vi "EventHandler-String Input with Prompt.vi"(6 "Font":T2={"Normal-Font"={"Name"="Application Font", "Italic"=FALSE, "Color"=0, "Bold"=FALSE, "Size"=17}, "Prompt-Font"={"Name"="Application Font", "Italic"=TRUE, "Color"=3381759, "Bold"=FALSE, "Size"=15}}, 8 "Error in":errorcluster caption="Error in (no error)", 9 "Input Display Style":T1(ring), 10 "HintString":string, 11 "reference":refnum<vi>) -> (0 "Error out":errorcluster, 3 "reference (dup)":refnum<vi>)   [LabVIEW 2017]
doc: "Event handler that shows HintString as a prompt inside a string control until the user types, and shows it again when the field is left empty. The font and input display style of the control are configurable."
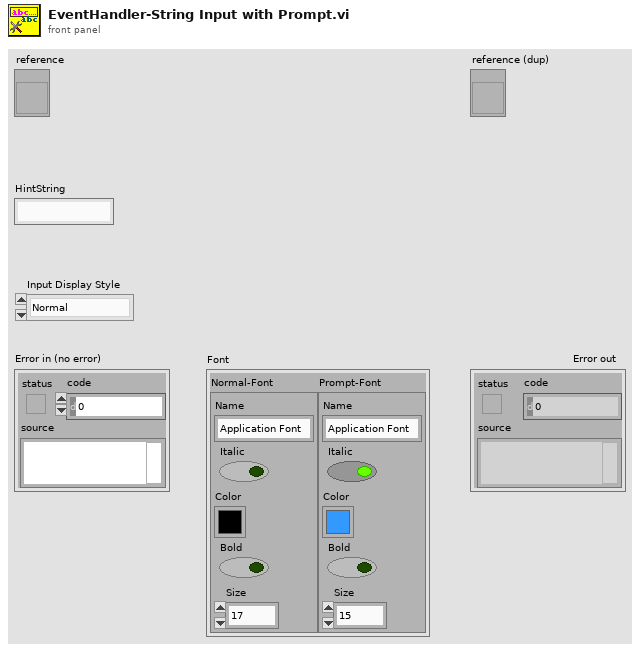
[diagram p1: front panel]
types:
  T1 = enum16{"Normal", "Backslash \"\\\"", "Password", "HEX"}
  T2 = cluster{"Normal-Font":cluster{"Name":string, "Italic":bool, "Color":u32, "Bold":bool, "Size":i32}, "Prompt-Font":cluster{"Name":string, "Italic":bool, "Color":u32, "Bold":bool, "Size":i32}}
  T3 = cluster{"Name":string, "Italic":bool, "Color":u32, "Bold":bool, "Size":i32}
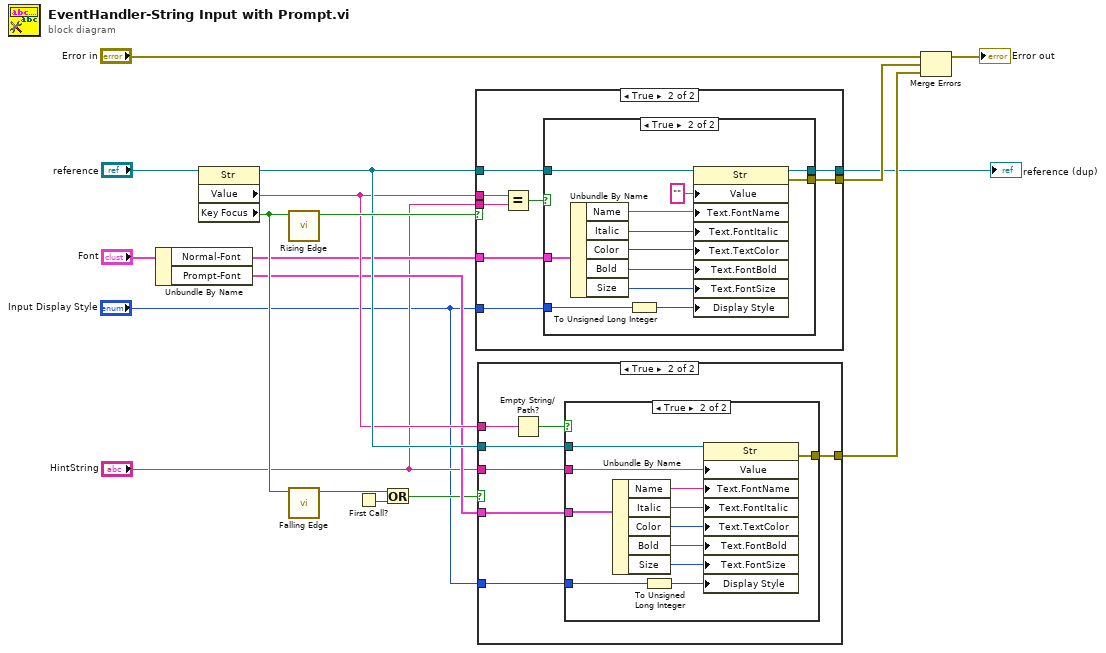
[diagram p0: block diagram]
diagram:
  n1 = Unbundle By Name("Font") -> ("Normal-Font"=w11:T3, "Prompt-Font"=w10:T3)
  n2 = property class="Str"(reference="reference") -> (reference out=w13:refnum<vi>, "Value"=w12:string, "Key Focus"=w17:bool)  [unwired: 1 in, 1 out]
  n3 = call "Rising Edge.vi"("signal"=w17) -> ("rising edge"=w16:bool)  [unwired: 10 in]
  n4 = call "Falling Edge.vi"("signal"=w17) -> ("falling edge"=w14:bool)  [unwired: 10 in]
  n5 = First Call?() -> (First Call?: T/F=w2:bool)
  n6 = Or(x=w14, y=w2) -> (x .or. y?=w3:bool)
  n7 = case shown="True" w16 {
    tunnel: w13 -> [w19 w27]
    tunnel: w12 -> [_ w25]
    tunnel: w11 -> [_ w23]
    tunnel: "HintString" -> [_ w24]
    tunnel: "Input Display Style" -> [_ w22]
    tunnel: [_ w21] -> w6
    tunnel: [w19 w20] -> w4
    frame False {
    }
    frame True {
      n8 = Equal?(x=w25, y=w24) -> (x = y?=w26:bool)
      n9 = case shown="True" w26 {
        tunnel: w27 -> [w28 w39]
        tunnel: w23 -> [_ w40]
        tunnel: w22 -> [_ w32]
        tunnel: [_ w31] -> w21
        tunnel: [w28 w30] -> w20
        frame False {
        }
        frame True {
          n10 = Unbundle By Name(w40) -> ("Name"=w38:string, "Italic"=w37:bool, "Color"=w36:u32, "Bold"=w35:bool, "Size"=w34:i32)
          n11 = To Unsigned Long Integer(number=w32) -> (unsigned 32bit integer=w29:u32)
          n12 = property class="Str"(reference=w39, "Value"="", "Text.FontName"=w38, "Text.FontItalic"=w37, "Text.TextColor"=w36, "Text.FontBold"=w35, "Text.FontSize"=w34, "Display Style"=w29) -> (reference out=w30:refnum<vi>, error out=w31:errorcluster)  [unwired: 1 in]
        }
      }
    }
  }
  "reference (dup)" <- w4
  n13 = case shown="True" w3 {
    tunnel: w13 -> [_ w47]
    tunnel: w12 -> [_ w46]
    tunnel: w10 -> [_ w44]
    tunnel: "HintString" -> [_ w43]
    tunnel: [_ w42] -> w5
    tunnel: "Input Display Style" -> [_ w41]
    frame False {
    }
    frame True {
      n14 = Empty String/Path?(string/path=w46) -> (empty?=w45:bool)
      n15 = case shown="True" w45 {
        tunnel: w47 -> [_ w58]
        tunnel: w44 -> [_ w57]
        tunnel: w43 -> [_ w51]
        tunnel: [_ w50] -> w42
        tunnel: w41 -> [_ w49]
        frame False {
        }
        frame True {
          n16 = Unbundle By Name(w57) -> ("Name"=w56:string, "Italic"=w55:bool, "Color"=w54:u32, "Bold"=w53:bool, "Size"=w52:i32)
          n17 = To Unsigned Long Integer(number=w49) -> (unsigned 32bit integer=w48:u32)
          n18 = property class="Str"(reference=w58, "Value"=w51, "Text.FontName"=w56, "Text.FontItalic"=w55, "Text.TextColor"=w54, "Text.FontBold"=w53, "Text.FontSize"=w52, "Display Style"=w48) -> (error out=w50:errorcluster)  [unwired: 1 in, 1 out]
        }
      }
    }
  }
  n19 = Merge Errors("Error in", w6, w5) -> (→"Error out":errorcluster)
